vi "TIFKATS Controller.vi"(8 "error in":errorcluster) -> ()   [LabVIEW 2023]
doc: "This VI executes continuously carrying out the current operation and responding to updates or new operations. It will often contain the timing or control code that is difficult to place directly in TeleOp. This VI generally opens all sensors and motors and isolates the rest of the robot code from knowing how the operations are carried out."
uses:
  <vilib>/Rock Robotics/WPI/Framework/Completion Status.ctl
  TIFKATS Setpoints2b.ctl
  TIFKATS Operations.ctl
  <vilib>/Rock Robotics/WPI/ThirdParty/REV Robotics/REVLib/Typedef/Spark MAX Control Type.ctl
  <vilib>/Rock Robotics/Network Tables/NT Write Boolean.vi
panel:
  in  "Interactive Values":T1
  out "Current\nCmd":string="Started at  16:06:33.078\nDefault: Immediate,  S 2.0, D 0.000000"
  in  "Buttons":cluster{"Execute Cmd":bool, "Abort Cmd":bool}
  out "Command Timing":cluster{"Start Time (ms)":u32, "Iterations":i32}={"Start Time (ms)"=10304663, "Iterations"=0}
  out "Status":T3
  # "Tip: It may be helpful to observe inputs and sensor values.\nYou may also want to display tuning or debugging controls."
  # "Interactive Command: You may fill in the settings for a command\nand schedule it with the Execute button. You can observe and abort\nany command while fine tuning the code for the controller."
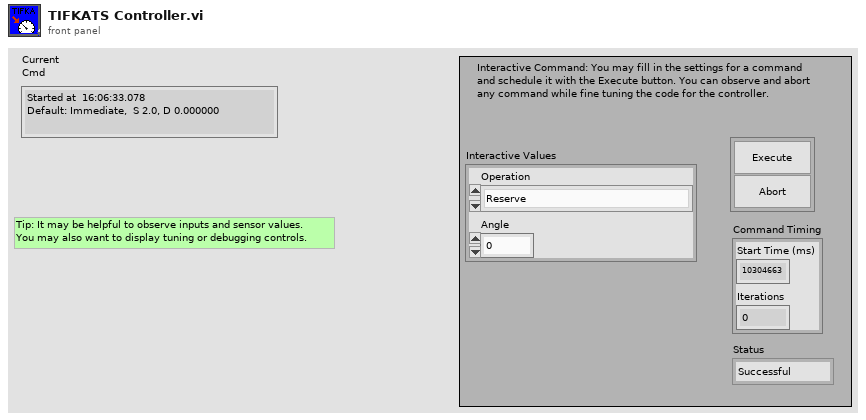
[diagram p1: front panel]
types:
  T1 = typedef "TIFKATS Setpoints2b.ctl" = cluster{"Operation":T2, "Angle":dbl}
  T2 = typedef "TIFKATS Operations.ctl" = enum16{"Reserve", "Read Current", "Immediate", "Load", "Shoot", "Intake", "Spit", "Stop All"}
  T3 = typedef "Completion Status.ctl" = enum16{"Successful", "Aborted", "Incomplete"}
  T4 = typedef "Command Status Info.ctl" = cluster{"Name":string, "Status":T3, "notifier out":T5}
  T5 = typedef "Completion Notifier.ctl" = refnum<notifier>
  T6 = cluster{"Current Command":T1, "Command Timing":cluster{"Start Time (ms)":u32, "Iterations":i32}, "Command Arguments":cluster{"Command Info":T4, "Description":string, "Default Command":T1, "queue out":refnum<queue>, "Subsystem Name":string}}
  T7 = typedef "Spark MAX Control Type.ctl" = enum16{"Percent VBus", "Voltage", "Velocity", "Position", "Smart Motion", "Current", "Smart Velocity"}
  T8 = typedef "WPI_MotorControlDeviceRef.ctl" = cluster{"DeviceStatus":errorcluster, "Type":T9, "PWM":cluster{"PWM Channel":T10, "DeadBand":T11}, "CAN":cluster{"Device Number":u8, "SetOutput VI Ref":variant, "GetOutput VI Ref":variant, "Enable VI Ref":variant, "Disable VI Ref":variant, "Data":variant}, "Invert":bool, "DIO PWM":cluster{"PWM \"Enable\" Channel":T10, "DIOChannel":T12, "PWM Rate":dbl}}
  T9 = typedef "WPI_MotorControlType.ctl" = enum16{"PWM", "CAN", "DIO PWM"}
  T10 = typedef "FPGA_DIOPWMChannel.ctl" = enum8{"PWM 0", "PWM 1", "PWM 2", "PWM 3", "PWM 4", "PWM 5", "PWM 6", "PWM 7", "PWM 8", "PWM 9", "PWM MXP 0", "PWM MXP 1", "PWM MXP 2", "PWM MXP 3", "PWM MXP 4", "PWM MXP 5", "PWM MXP 6", "PWM MXP 7", "PWM MXP 8", "PWM MXP 9", "Invalid"}
  T11 = typedef "WPI_PWMDeadband.ctl" = cluster{"Name":string, "maxPositivePwm":i32, "minPositivePwm":i32, "centerPwm":i32, "maxNegativePwm":i32, "minNegativePwm":i32, "angularRange":u16}
  T12 = typedef "FPGA_DIOChannel.ctl" = enum8{"DIO 0", "DIO 1", "DIO 2", "DIO 3", "DIO 4", "DIO 5", "DIO 6", "DIO 7", "DIO 8", "DIO 9", "DIO MXP 0", "DIO MXP 1", "DIO MXP 2", "DIO MXP 3", "DIO MXP 4", "DIO MXP 5", "DIO MXP 6", "DIO MXP 7", "DIO MXP 8", "DIO MXP 9", "DIO MXP 10", "DIO MXP 11", "DIO MXP 12", "DIO MXP 13", "DIO MXP 14", "DIO MXP 15", "SPI Port CS1", "SPI Port CS2", "SPI Port CS3", "SPI Port MISO", "SPI Port MOSI", "Invalid"}
  T13 = typedef "WPI_DigitalInputDevRef.ctl" = cluster{"DevStatus":errorcluster, "DIO Channel":T12}
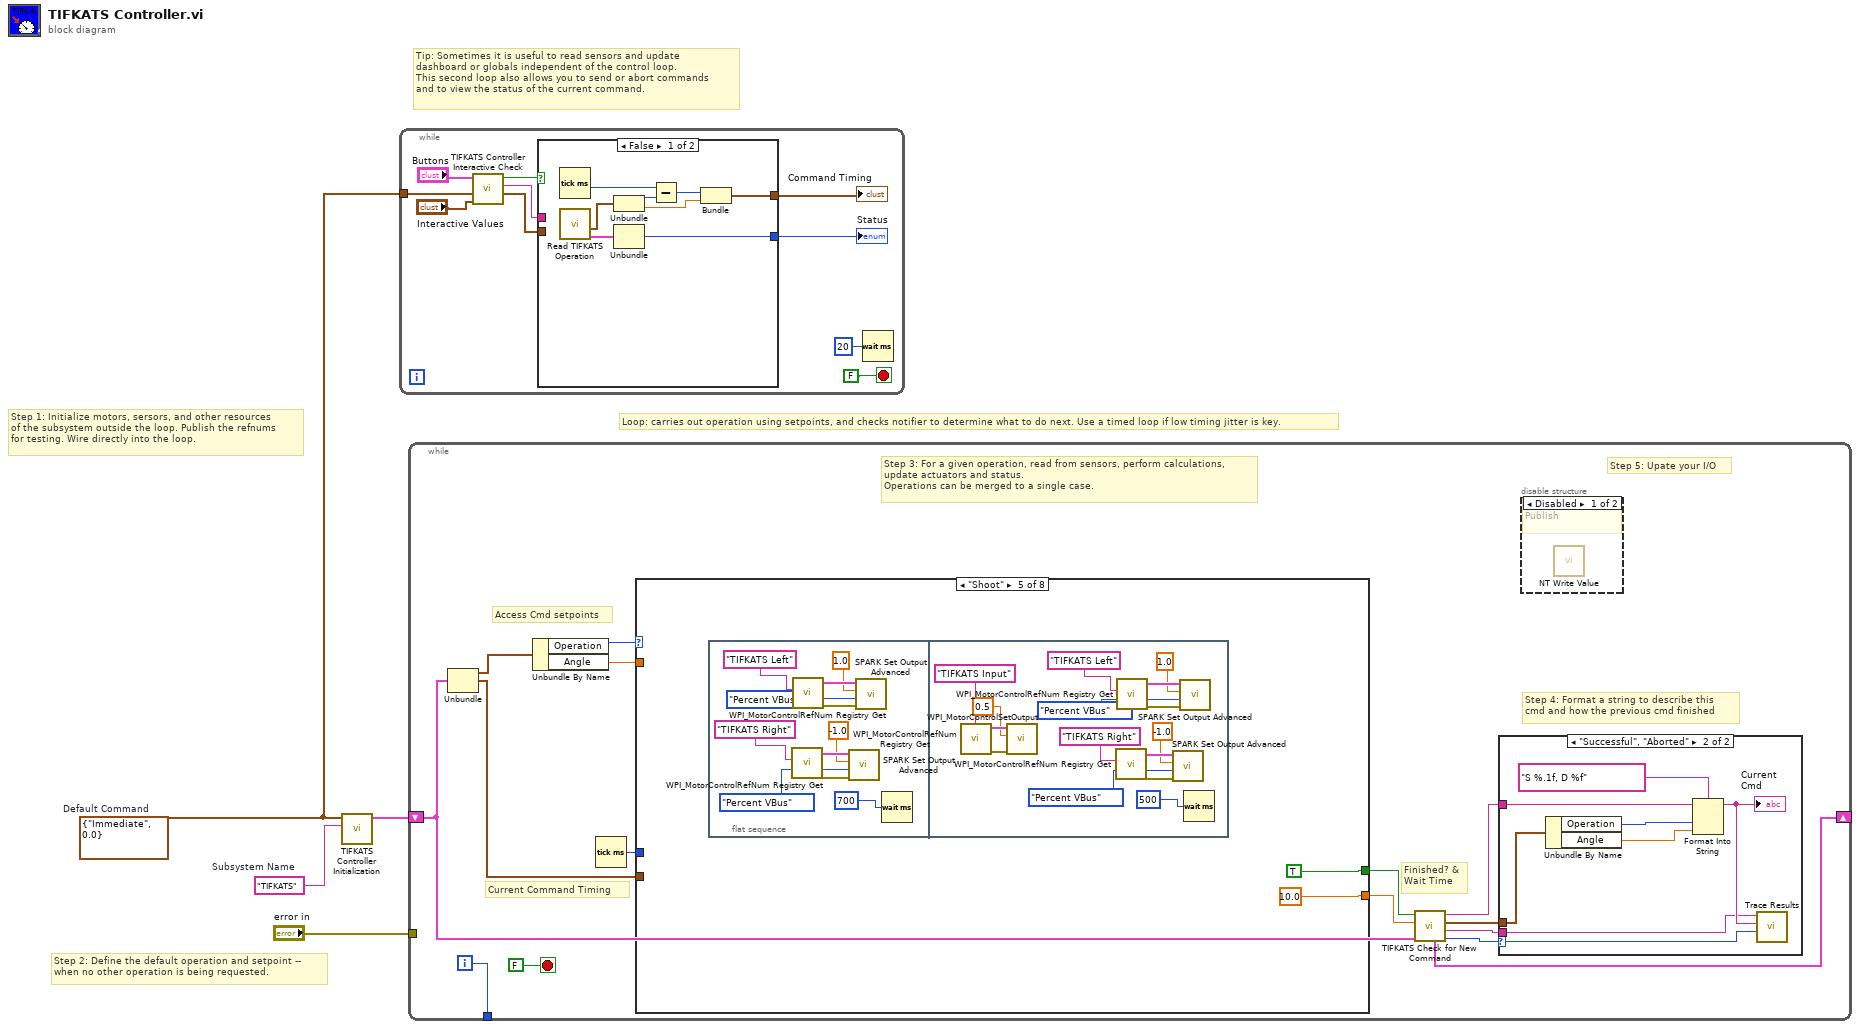
[diagram p0: block diagram]
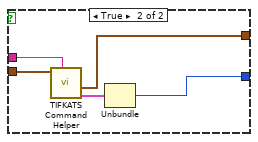
[diagram p2: hidden frame]
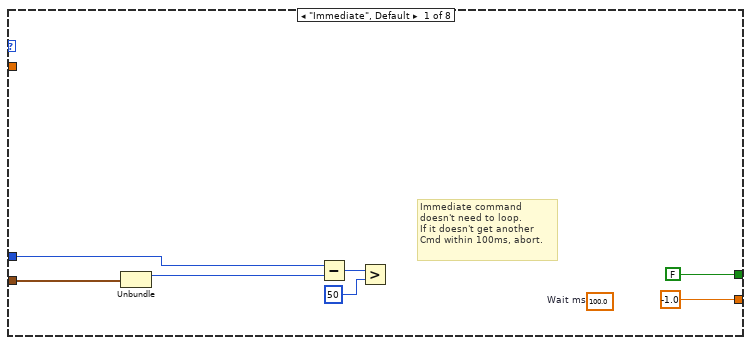
[diagram p5: hidden frame]
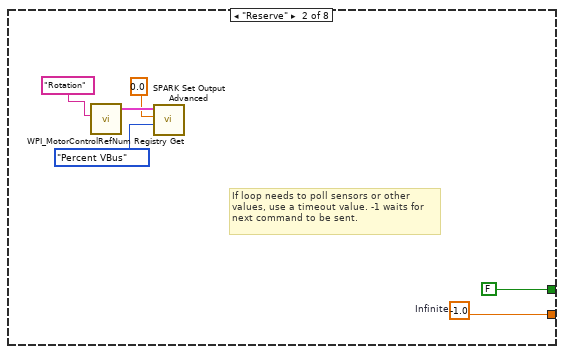
[diagram p6: hidden frame]
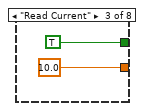
[diagram p7: hidden frame]
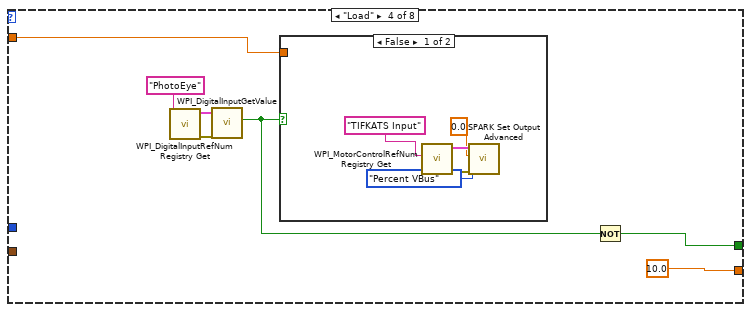
[diagram p8: hidden frame]
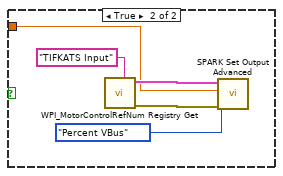
[diagram p9: hidden frame]
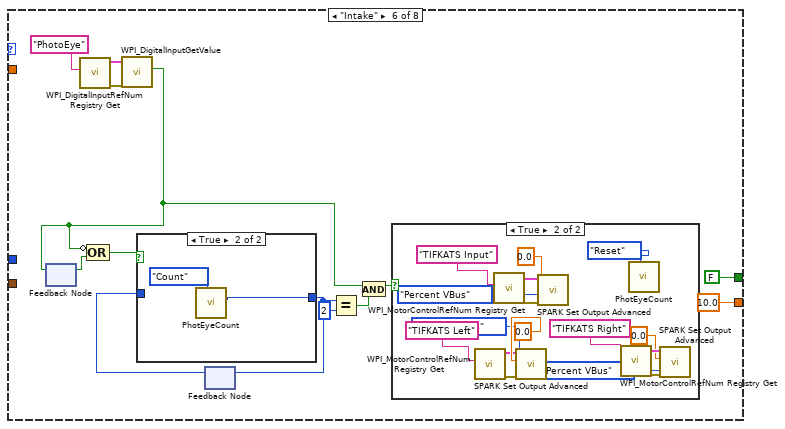
[diagram p10: hidden frame]
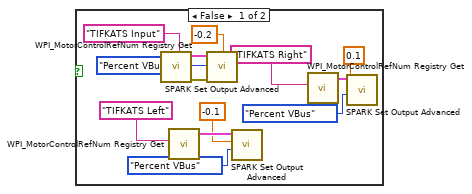
[diagram p11: hidden frame]
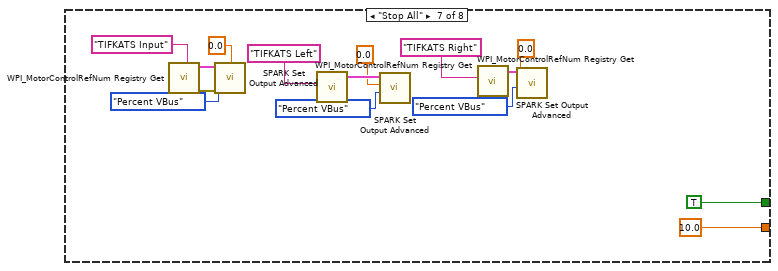
[diagram p13: hidden frame]
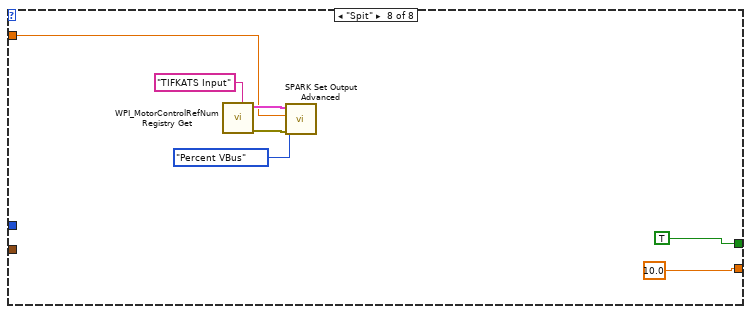
[diagram p14: hidden frame]
diagram:
  w1 = T1 {"Operation"=enum."Immediate", "Angle"=0.0}  # Default Command
  w2 = "TIFKATS"  # Subsystem Name
  # "Tip: Sometimes it is useful to read sensors and update\ndashboard or globals independent of the control loop.\nThis second loop also allows you to send or abort commands\nand to view the status of the current command."
  # "Step 2: Define the default operation and setpoint --\nwhen no other operation is being requested."
  # "Step 1: Initialize motors, sersors, and other resources\nof the subsystem outside the loop. Publish the refnums\nfor testing. Wire directly into the loop."
  # "Loop: carries out operation using setpoints, and checks notifier to determine what to do next. Use a timed loop if low timing jitter is key."
  n1 = call "TIFKATS Controller Initialization.vi"("Subsystem Name"=w2, "Default Command"=w1) -> ("Current Command"=w3:T6)  [unwired: 9 in]
  n2 = while {
    tunnel: w1 -> [w11]
    stop <- FALSE stop-if-true
    n3 = call "TIFKATS Controller Interactive Check.vi"("Interactive Command in"="Interactive Values", "Default Command"=w11, "Buttons"="Buttons") -> ("Interactive Command out"=w8:T1, "Trace String"=w9:string, "Schedule"=w10:bool)  [unwired: 6 in]
    n4 = case shown="False" w10 {
      tunnel: [w22 w27] -> w7
      tunnel: w8 -> [_ w25]
      tunnel: [w18 w23] -> w6
      tunnel: w9 -> [_ w26]
      frame False {
        n5 = Tick Count (ms)() -> (millisecond timer value=w17:u32)
        n6 = call "Read TIFKATS Operation.vi"() -> ("Command Info"=w15:T4, "SubSystem Data"=w16:T1)  [unwired: 9 in, 1 out]
        n7 = Unbundle(w16) -> ("Operation"=w21:T2, "Angle"=w19:dbl)
        n8 = Unbundle(w15) -> ("Status"=w22:T3)  [unwired: 2 out]
        n9 = Subtract(x=w17, y=w21) -> (x-y=w20:u32)
        n10 = Bundle(w20, "Angle"=w19) -> (w18:cluster{u32, "Angle":dbl})  [unwired: 1 in]
      }
      frame True {
        n11 = call "TIFKATS Command Helper.vi"("Description"=w26, "SubSystem Data"=w25) -> ("Command Info Out"=w24:T4, "Command Timing"=w23:cluster{"Start Time (ms)":u32, "Iterations":i32})  [unwired: 7 in, 1 out]
        n12 = Unbundle(w24) -> ("Status"=w27:T3)  [unwired: 2 out]
      }
    }
    "Status" <- w7
    "Command Timing" <- w6
    n13 = Wait (ms)(milliseconds to wait=u32 20) -> ()  [unwired: 1 out]
  }
  n14 = while {
    shift-right: [w35] -> _
    shift-left: w3 -> [w28]
    tunnel: [w41] -> _
    tunnel: "error in" -> [_]
    i -> [w41]
    stop <- FALSE stop-if-true
    # "Step 5: Upate your I/O"
    # "Step 4: Format a string to describe this\ncmd and how the previous cmd finished"
    # "Current Command Timing"
    # "Access Cmd setpoints"
    # "Finished? &\nWait Time"
    # "Step 3: For a given operation, read from sensors, perform calculations,\nupdate actuators and status.\nOperations can be merged to a single case."
    n15 = Unbundle(w28) -> ("Current Command"=w40:T1, "Command Timing"=w36:cluster{"Start Time (ms)":u32, "Iterations":i32})  [unwired: 1 out]
    n16 = Unbundle By Name(w40) -> ("Operation"=w39:T2, "Angle"=w38:dbl)
    n17 = Tick Count (ms)() -> (millisecond timer value=w37:u32)
    n18 = case shown="\"Shoot\"" w39 {
      tunnel: [-1.0 ("Infinite") w63 10.0 ("Infinite") 10.0 ("Infinite") 10.0 ("Infinite") 10.0 ("Infinite") 10.0 ("Infinite") 10.0 ("Infinite")] -> w33
      tunnel: [FALSE ("ignore previous (F)") FALSE ("ignore previous (F)") TRUE ("ignore previous (F)") w66 TRUE ("ignore previous (F)") FALSE ("ignore previous (F)") TRUE ("ignore previous (F)") TRUE ("ignore previous (F)")] -> w34
      tunnel: w36 -> [w54 _ _ _ _ _ _ _]
      tunnel: w38 -> [_ _ _ w68 _ _ _ w171]
      tunnel: w37 -> [w53 _ _ _ _ _ _ _]
      frame "Immediate", Default {
        (unwired) 100.0  # Wait ms
        # "Immediate command\ndoesn't need to loop.\nIf it doesn't get another\nCmd within 100ms, abort."
        n19 = Unbundle(w54) -> ("Start Time (ms)"=w57:u32)  [unwired: 1 out]
        n20 = Subtract(x=w53, y=w57) -> (x-y=w56:u32)
        n21 = Greater?(x=w56, y=u8 50 ("Left Motor")) -> ()  [unwired: 1 out]
      }
      frame "Reserve" {
        w63 = -1.0  # Infinite
        # "If loop needs to poll sensors or other\nvalues, use a timeout value. -1 waits for\nnext command to be sent."
        n22 = call <vilib>:"WPI_MotorControlRefNum Registry Get.vi"("refnum name"="Rotation") -> ("MotorControlDevRef"=w60:T8)  [unwired: 9 in, 1 out]
        n23 = call <vilib>:"SPARK Set Output Advanced.vi"("Control Mode"=Spark_MAX_Control_Type."Percent VBus", "Setpoint"=0.0 ("Output"), "MotorControlDevRef"=w60) -> ()  [unwired: 7 in, 2 out]
      }
      frame "Read Current" {
      }
      frame "Load" {
        n24 = call <vilib>:"WPI_DigitalInputRefNum Registry Get.vi"("refnum name"="PhotoEye") -> ("error out"=w71:errorcluster, "DigitalInputDevRef"=w70:T13)  [unwired: 9 in]
        n25 = call <vilib>:"WPI_DigitalInputGetValue.vi"("error in (no error)"=w71, "DigitalInputDevRef"=w70) -> ("Value"=w67:bool)  [unwired: 7 in, 2 out]
        n26 = case shown="False" w67 {
          tunnel: w68 -> [_ w78]
          frame False {
            n27 = call <vilib>:"WPI_MotorControlRefNum Registry Get.vi"("refnum name"="TIFKATS Input") -> ("error out"=w75:errorcluster, "MotorControlDevRef"=w76:T8)  [unwired: 9 in]
            n28 = call <vilib>:"SPARK Set Output Advanced.vi"("error in (no error)"=w75, "Control Mode"=Spark_MAX_Control_Type."Percent VBus", "Setpoint"=0.0, "MotorControlDevRef"=w76) -> ()  [unwired: 6 in, 2 out]
          }
          frame True {
            n29 = call <vilib>:"WPI_MotorControlRefNum Registry Get.vi"("refnum name"="TIFKATS Input") -> ("error out"=w82:errorcluster, "MotorControlDevRef"=w81:T8)  [unwired: 9 in]
            n30 = call <vilib>:"SPARK Set Output Advanced.vi"("error in (no error)"=w82, "Control Mode"=Spark_MAX_Control_Type."Percent VBus", "Setpoint"=w78, "MotorControlDevRef"=w81) -> ()  [unwired: 6 in, 2 out]
          }
        }
        n31 = Not(x=w67) -> (.not. x?=w66:bool)
      }
      frame "Shoot" {
        n32 = flat-sequence {
          frame #0 {
            n33 = call <vilib>:"WPI_MotorControlRefNum Registry Get.vi"("refnum name"="TIFKATS Right") -> ("error out"=w85:errorcluster, "MotorControlDevRef"=w90:T8)  [unwired: 9 in]
            n34 = call <vilib>:"WPI_MotorControlRefNum Registry Get.vi"("refnum name"="TIFKATS Left") -> ("error out"=w86:errorcluster, "MotorControlDevRef"=w92:T8)  [unwired: 9 in]
            n35 = call <vilib>:"SPARK Set Output Advanced.vi"("error in (no error)"=w85, "Control Mode"=Spark_MAX_Control_Type."Percent VBus", "Setpoint"=-1.0 ("Output"), "MotorControlDevRef"=w90) -> ()  [unwired: 6 in, 2 out]
            n36 = call <vilib>:"SPARK Set Output Advanced.vi"("error in (no error)"=w86, "Control Mode"=Spark_MAX_Control_Type."Percent VBus", "Setpoint"=1.0 ("Output"), "MotorControlDevRef"=w92) -> ()  [unwired: 6 in, 2 out]
            n37 = Wait (ms)(milliseconds to wait=u32 700) -> ()  [unwired: 1 out]
          }
          frame #1 {
            n38 = call <vilib>:"WPI_MotorControlRefNum Registry Get.vi"("refnum name"="TIFKATS Input") -> ("error out"=w109:errorcluster, "MotorControlDevRef"=w110:T8)  [unwired: 9 in]
            n39 = call <vilib>:"WPI_MotorControlSetOutput.vi"("error in (no error)"=w109, "Output"=0.5, "MotorControlDevRef"=w110) -> ()  [unwired: 6 in, 3 out]
            n40 = call <vilib>:"WPI_MotorControlRefNum Registry Get.vi"("refnum name"="TIFKATS Right") -> ("error out"=w98:errorcluster, "MotorControlDevRef"=w102:T8)  [unwired: 9 in]
            n41 = call <vilib>:"WPI_MotorControlRefNum Registry Get.vi"("refnum name"="TIFKATS Left") -> ("error out"=w99:errorcluster, "MotorControlDevRef"=w104:T8)  [unwired: 9 in]
            n42 = call <vilib>:"SPARK Set Output Advanced.vi"("error in (no error)"=w98, "Control Mode"=Spark_MAX_Control_Type."Percent VBus", "Setpoint"=-1.0 ("Output"), "MotorControlDevRef"=w102) -> ()  [unwired: 6 in, 2 out]
            n43 = call <vilib>:"SPARK Set Output Advanced.vi"("error in (no error)"=w99, "Control Mode"=Spark_MAX_Control_Type."Percent VBus", "Setpoint"=1.0 ("Output"), "MotorControlDevRef"=w104) -> ()  [unwired: 6 in, 2 out]
            n44 = Wait (ms)(milliseconds to wait=u32 500) -> ()  [unwired: 1 out]
          }
        }
      }
      frame "Intake" {
        n45 = feedback #1() -> (w118:bool)  [unwired: 1 in]
        n46 = call <vilib>:"WPI_DigitalInputRefNum Registry Get.vi"("refnum name"="PhotoEye") -> ("error out"=w123:errorcluster, "DigitalInputDevRef"=w122:T13)  [unwired: 9 in]
        n47 = call <vilib>:"WPI_DigitalInputGetValue.vi"("error in (no error)"=w123, "DigitalInputDevRef"=w122) -> ("Value"=w115:bool)  [unwired: 7 in, 2 out]
        n48 = feedback-in #1(w115) -> ()
        n49 = Compound Arithmetic op=OR(invert w115, w118) -> (w117:bool)
        n50 = feedback #2() -> (w116:i32)  [unwired: 1 in]
        n51 = case shown="True" w117 {
          tunnel: [w153 w154] -> w112
          tunnel: w116 -> [w153 _]
          frame False {
          }
          frame True {
            n52 = call "PhotEyeCount.vi"("Enum"=enum16{"Count", "Reset"}."Count") -> ("count"=w154:i32)  [unwired: 10 in]
          }
        }
        n53 = feedback-in #2(w112) -> ()
        n54 = Equal?(x=w112, y=2) -> (x = y?=w113:bool)
        n55 = And(x=w115, y=w113) -> (x .and. y?=w114:bool)
        n56 = case shown="True" w114 {
          frame False {
            n57 = call <vilib>:"WPI_MotorControlRefNum Registry Get.vi"("refnum name"="TIFKATS Input") -> ("error out"=w134:errorcluster, "MotorControlDevRef"=w133:T8)  [unwired: 9 in]
            n58 = call <vilib>:"WPI_MotorControlRefNum Registry Get.vi"("refnum name"="TIFKATS Left") -> ("MotorControlDevRef"=w135:T8)  [unwired: 9 in, 1 out]
            n59 = call <vilib>:"SPARK Set Output Advanced.vi"("error in (no error)"=w134, "Control Mode"=Spark_MAX_Control_Type."Percent VBus", "Setpoint"=-0.2 ("Output"), "MotorControlDevRef"=w133) -> ()  [unwired: 6 in, 2 out]
            n60 = call <vilib>:"SPARK Set Output Advanced.vi"("Control Mode"=Spark_MAX_Control_Type."Percent VBus", "Setpoint"=-0.1 ("Output"), "MotorControlDevRef"=w135) -> ()  [unwired: 7 in, 2 out]
            n61 = call <vilib>:"WPI_MotorControlRefNum Registry Get.vi"("refnum name"="TIFKATS Right") -> ("MotorControlDevRef"=w136:T8)  [unwired: 9 in, 1 out]
            n62 = call <vilib>:"SPARK Set Output Advanced.vi"("Control Mode"=Spark_MAX_Control_Type."Percent VBus", "Setpoint"=0.1 ("Output"), "MotorControlDevRef"=w136) -> ()  [unwired: 7 in, 2 out]
          }
          frame True {
            n63 = call <vilib>:"WPI_MotorControlRefNum Registry Get.vi"("refnum name"="TIFKATS Left") -> ("error out"=w141:errorcluster, "MotorControlDevRef"=w146:T8)  [unwired: 9 in]
            n64 = call <vilib>:"WPI_MotorControlRefNum Registry Get.vi"("refnum name"="TIFKATS Input") -> ("error out"=w142:errorcluster, "MotorControlDevRef"=w143:T8)  [unwired: 9 in]
            n65 = call <vilib>:"SPARK Set Output Advanced.vi"("error in (no error)"=w141, "Control Mode"=Spark_MAX_Control_Type."Percent VBus", "Setpoint"=0.0 ("Output"), "MotorControlDevRef"=w146) -> ()  [unwired: 6 in, 2 out]
            n66 = call <vilib>:"SPARK Set Output Advanced.vi"("error in (no error)"=w142, "Control Mode"=Spark_MAX_Control_Type."Percent VBus", "Setpoint"=0.0 ("Output"), "MotorControlDevRef"=w143) -> ()  [unwired: 6 in, 2 out]
            n67 = call <vilib>:"WPI_MotorControlRefNum Registry Get.vi"("refnum name"="TIFKATS Right") -> ("error out"=w140:errorcluster, "MotorControlDevRef"=w149:T8)  [unwired: 9 in]
            n68 = call "PhotEyeCount.vi"("Enum"=enum16{"Count", "Reset"}."Reset") -> ()  [unwired: 10 in, 1 out]
            n69 = call <vilib>:"SPARK Set Output Advanced.vi"("error in (no error)"=w140, "Control Mode"=Spark_MAX_Control_Type."Percent VBus", "Setpoint"=0.0 ("Output"), "MotorControlDevRef"=w149) -> ()  [unwired: 6 in, 2 out]
          }
        }
      }
      frame "Stop All" {
        n70 = call <vilib>:"WPI_MotorControlRefNum Registry Get.vi"("refnum name"="TIFKATS Input") -> ("error out"=w168:errorcluster, "MotorControlDevRef"=w167:T8)  [unwired: 9 in]
        n71 = call <vilib>:"SPARK Set Output Advanced.vi"("error in (no error)"=w168, "Control Mode"=Spark_MAX_Control_Type."Percent VBus", "Setpoint"=0.0 ("Output"), "MotorControlDevRef"=w167) -> ()  [unwired: 6 in, 2 out]
        n72 = call <vilib>:"WPI_MotorControlRefNum Registry Get.vi"("refnum name"="TIFKATS Left") -> ("MotorControlDevRef"=w169:T8)  [unwired: 9 in, 1 out]
        n73 = call <vilib>:"SPARK Set Output Advanced.vi"("Control Mode"=Spark_MAX_Control_Type."Percent VBus", "Setpoint"=0.0 ("Output"), "MotorControlDevRef"=w169) -> ()  [unwired: 7 in, 2 out]
        n74 = call <vilib>:"WPI_MotorControlRefNum Registry Get.vi"("refnum name"="TIFKATS Right") -> ("MotorControlDevRef"=w170:T8)  [unwired: 9 in, 1 out]
        n75 = call <vilib>:"SPARK Set Output Advanced.vi"("Control Mode"=Spark_MAX_Control_Type."Percent VBus", "Setpoint"=0.0 ("Output"), "MotorControlDevRef"=w170) -> ()  [unwired: 7 in, 2 out]
      }
      frame "Spit" {
        n76 = call <vilib>:"WPI_MotorControlRefNum Registry Get.vi"("refnum name"="TIFKATS Input") -> ("error out"=w175:errorcluster, "MotorControlDevRef"=w174:T8)  [unwired: 9 in]
        n77 = call <vilib>:"SPARK Set Output Advanced.vi"("error in (no error)"=w175, "Control Mode"=Spark_MAX_Control_Type."Percent VBus", "Setpoint"=w171, "MotorControlDevRef"=w174) -> ()  [unwired: 6 in, 2 out]
      }
    }
    n78 = call "TIFKATS Check for New Command.vi"("Current Command"=w28, "Wait time (ms)"=w33, "Finished?"=w34) -> ("Completion"=w29:T3, "Subsystem Name"=w30:string, "Current Command"=w31:T1, "Initial Trace String"=w32:string, "NextCommand"=w35:T6)  [unwired: 4 in]
    n79 = case shown="\"Successful\", \"Aborted\"" w29 {
      selector: w29 -> [_ w50]
      tunnel: w32 -> [_ w46]
      tunnel: w31 -> [_ w47]
      tunnel: w30 -> [_ w43]
      frame "Incomplete", Default {
        # "Continuing current command"
      }
      frame "Successful", "Aborted" {
        # "Report and setup for next command"
        n80 = Unbundle By Name(w47) -> ("Operation"=w49:T2, "Angle"=w44:dbl)
        n81 = Format Into String(format string="S %.1f, D %f", initial string=w46, w49, w44) -> (resulting string=w45:string)  [unwired: 1 in, 1 out]
        "Current\nCmd" <- w45
        n82 = call <vilib>:"Trace Results.vi"("Status of previous command"=w50, "Description"=w45, "Subsystem"=w43) -> ()  [unwired: 9 in]
      }
    }
    n83 = disable-structure shown="Disabled" {
      frame Disabled {
        # "Publish"
        n84 = call-poly <vilib>:"NT Write Value.vi"() -> ()  [unwired: 11 in, 1 out]
      }
      frame Enabled {
      }
    }
  }
